vi "acknowledgeIRQ.vi"(8 "error in (no error)":errorcluster, 10 "IRQs":i32[](array[numeric]), 11 "IIRQ in":refnum<class "IIRQ.lvclass">) -> (0 "error out":errorcluster, 3 "IIRQ out":refnum<class "IIRQ.lvclass">)   [LabVIEW 2016, in "RTFPGA.lvlib" / "IIRQ.lvclass"]
uses:
  IIRQ.lvclass
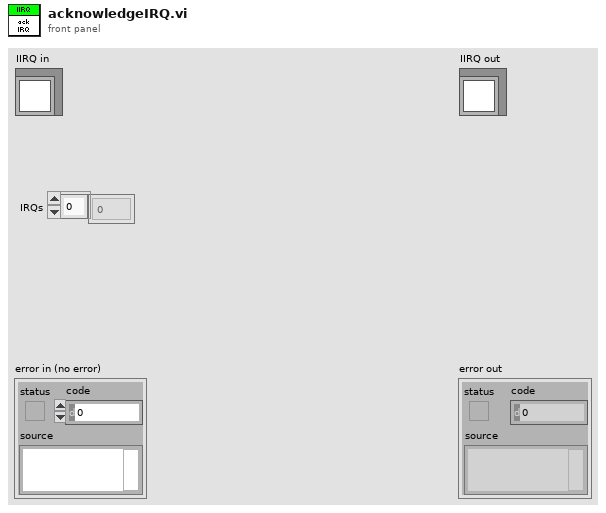
[diagram p1: front panel]
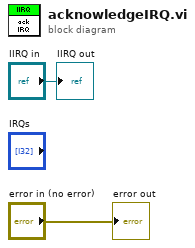
[diagram p0: block diagram]
diagram:
  "error out" <- "error in (no error)"
  "IIRQ out" <- "IIRQ in"
